vi "Result_Test.vi"(8 "error in (no error)":errorcluster caption="entrée d'erreur (pas d'erreur)", 11 "Get_Voltage en entrée":refnum<class "Wait_Frame_ERP1.lvclass">) -> (0 "error out":errorcluster caption="sortie d'erreur", 3 "Get_Voltage en sortie":refnum<class "Wait_Frame_ERP1.lvclass">)   [LabVIEW 2020, in "Library Test.lvlib" / "Wait_Frame_ERP1.lvclass"]
uses:
  Wait_Frame_ERP1.lvclass
  C:/Users/ngarcin/OneDrive - Altyor/Standard TB/Suite TB45/Class/Test/Test (Default)/Test (Default).lvclass
  Commun VI/TypeDef/Variable Printable.ctl
  Test_Wtih_Instr/Test_With_Inst.lvclass
  Commun VI/Library Commun.lvlib
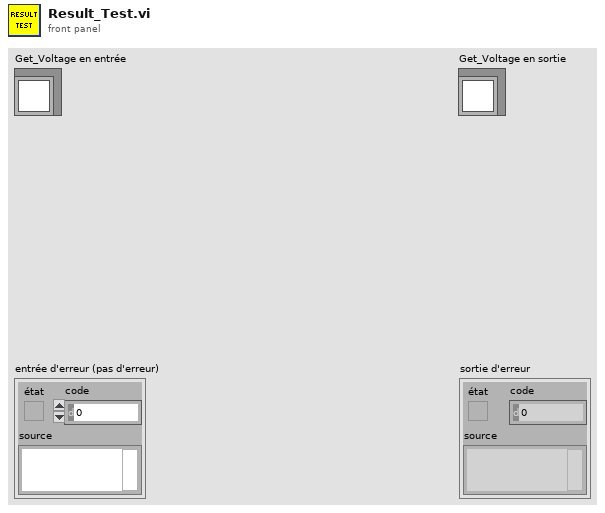
[diagram p1: front panel]
types:
  T1 = typedef "Variable Printable.ctl" = string
  T2 = enum16{"Get Variable", "Get All Variables", "Set Variable", "Delete Variable", "Delete All Variable"}
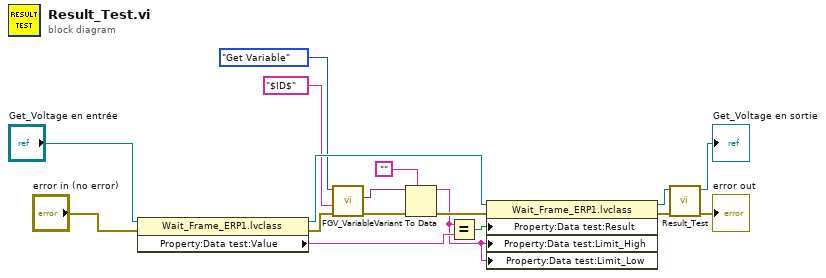
[diagram p0: block diagram]
diagram:
  n1 = property class="Wait_Frame_ERP1.lvclass"(reference="Get_Voltage en entrée", error in="error in (no error)") -> (reference out=w17:refnum<class "Wait_Frame_ERP1.lvclass">, error out=w3:errorcluster, "Property:Data test:Value"=w5:string)
  n2 = call "FGV_Variable.vi"("error in (no error)"=w3, "Variable"=T1 "$ID$", "Function"=T2."Get Variable") -> ("error out"=w8:errorcluster, "Data Out"=w6:variant)  [unwired: 6 in, 1 out]
  n3 = Variant To Data(error in=w8, type="", Variant=w6) -> (data=w1:string, error out=w2:errorcluster)
  n4 = Equal?(x=w1, y=w5) -> (x = y?=w4:bool)
  n5 = property class="Wait_Frame_ERP1.lvclass"(reference=w17, error in=w2, "Property:Data test:Result"=w4, "Property:Data test:Limit_High"=w1, "Property:Data test:Limit_Low"=w1) -> (reference out=w11:refnum<class "Wait_Frame_ERP1.lvclass">, error out=w14:errorcluster)
  n6 = call-parent "Result_Test.vi"("error in (no error)"=w14, "Test_With_Inst en entrée"=w11) -> ("error out"=→"error out":errorcluster, "Test_With_Inst en sortie"=→"Get_Voltage en sortie":refnum<class "Wait_Frame_ERP1.lvclass">)  [unwired: 8 in]
